vi "Cache Entity.vi"(8 "error in (no error)":errorcluster, 10 "Conditum:Entity":refnum<class "Entity.lvclass">, 11 "Unit Of Work in":refnum<class "Unit Of Work Session.lvclass">) -> (0 "error out":errorcluster)   [LabVIEW 2020, in "Conditum.lvlib" / "Unit Of Work Session.lvclass"]
uses:
  Unit Of Work Session.lvclass
  Unit Of Work Session.lvclass/Unit Of Work Session.ctl
  <vilib>/Utility/miscctls.llb/LVMapReplaceAction.ctl
  Entity/Entity.lvclass
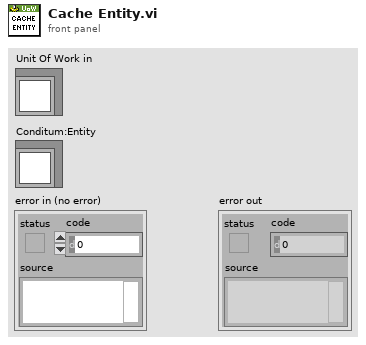
[diagram p1: front panel]
types:
  T1 = typedef "Conditum.lvlib/Entity State.ctl" = enum16{"New", "Managed", "Detached", "Removed"}
  T2 = typedef "Conditum.lvlib/Entity ID.ctl" = i64
  T3 = typedef "LVMapReplaceAction.ctl" = enum32{"Modify Entry only if found", "Add or Modify Entry", "Delete Entry"}
  T4 = typedef "Conditum.lvlib/Unit Of Work Session.lvclass/Ref Data.ctl" = cluster{"Entity Class Map":T5}
  T5 = typedef "Conditum.lvlib/Unit Of Work Session.lvclass/Entity Class Map.ctl" = map{string, map{T2, refnum<class "Entity.lvclass">}}
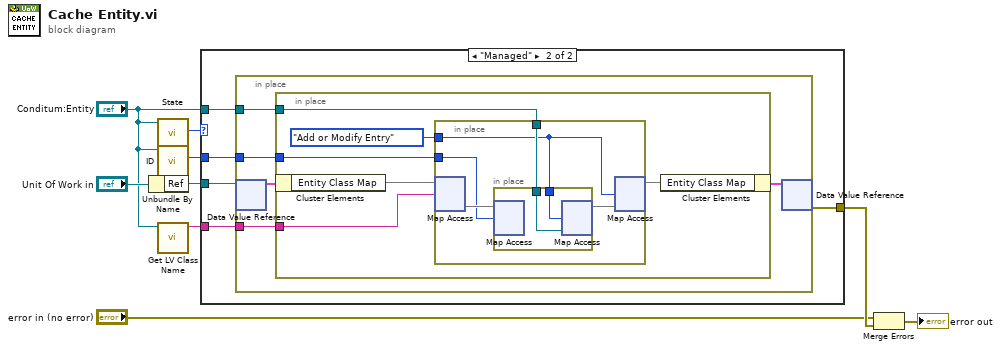
[diagram p0: block diagram]
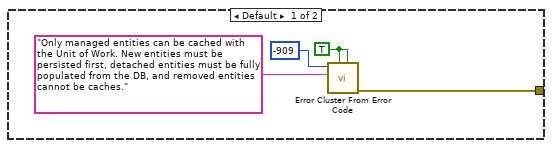
[diagram p2: hidden frame]
diagram:
  n1 = Unbundle By Name("Unit Of Work in") -> ("Ref"=w7:refnum<data-value>)
  n2 = call "State.vi"("Entity in"="Conditum:Entity") -> ("Entity State"=w1:T1)  [unwired: 10 in]
  n3 = call "ID.vi"("Entity in"="Conditum:Entity") -> ("ID"=w3:T2)  [unwired: 9 in, 1 out]
  n4 = call <vilib>:"Get LV Class Name.vi"("object"="Conditum:Entity") -> ("class name"=w9:string)  [unwired: 9 in, 1 out]
  n5 = case shown="\"Managed\"" w1 {
    tunnel: w9 -> [_ w18]
    tunnel: w7 -> [_ w17]
    tunnel: [w13 w16] -> w6
    tunnel: w3 -> [_ w15]
    tunnel: "Conditum:Entity" -> [_ w14]
    frame Default {
      w12 = TRUE ("is warning? (False)")
      n6 = call <vilib>:"Error Cluster From Error Code.vi"("is warning? (False)"=w12, "show call chain? (False)"=w12, "error message (\"\")"="Only managed entities can be cached with the Unit of Work. New entities must be persisted first, detached entities must be fully populated from the DB, and removed entities cannot be caches.", "error code (0)"=-909) -> ("error out"=w13:errorcluster)  [unwired: 5 in]
    }
    frame "Managed" {
      n7 = in-place {
        in-place-border: w18 -> [w22]
        in-place-border: w14 -> [w20]
        in-place-border: w15 -> [w19]
        n8 = in-place-dvr #1(w17) -> (w23:T4)  [unwired: 1 out]
        n9 = in-place {
          in-place-border: w22 -> [w25]
          in-place-border: w20 -> [w27]
          in-place-border: w19 -> [w24]
          n10 = in-place-cluster #2(w23) -> ("Entity Class Map"=w29:T5)
          n11 = in-place {
            in-place-border: w27 -> [w33]
            in-place-border: LVMapReplaceAction."Add or Modify Entry" ("action") -> [w32]
            in-place-border: w24 -> [w30]
            n12 = in-place-map #3(w29, w25) -> (w34:map{T2, refnum<class "Entity.lvclass">})  [unwired: 1 in, 1 out]
            n13 = in-place {
              in-place-border: w33 -> [w35]
              in-place-border: w32 -> [w36]
              n14 = in-place-map #4(w34, w30) -> ()  [unwired: 1 in, 2 out]
              n15 = in-place-map #4(w35, w36) -> (w31:map{T2, refnum<class "Entity.lvclass">})  [unwired: 2 out]
            }
            n16 = in-place-map #3(w31, w32) -> (w28:T5)  [unwired: 2 out]
          }
          n17 = in-place-cluster #2("Entity Class Map"=w28) -> (w21:T4)
        }
        n18 = in-place-dvr #1(w21) -> (w16:errorcluster)  [unwired: 1 out]
      }
    }
  }
  n19 = Merge Errors("error in (no error)", w6) -> (→"error out":errorcluster)
